vi "extract_force_data.vi"(11 "force_curve_data":dbl[][](array[numeric])) -> (3 "extracted_force_data":dbl[](array[numeric]))   [LabVIEW 2015]
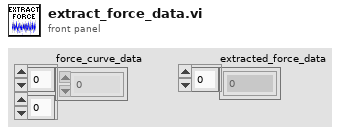
[diagram p1: front panel]
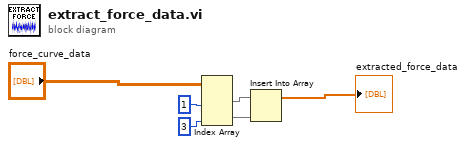
[diagram p0: block diagram]
diagram:
  n1 = Index Array(array="force_curve_data", index (col) #1=1 ("index (row)"), index (col) #2=3 ("index (col)")) -> (element #1=w4:dbl[], element #2=w5:dbl[])  [unwired: 2 in]
  n2 = Insert Into Array(array=w4, new element=w5) -> (→"extracted_force_data":dbl[])  [unwired: 1 in]
